vi "USRP Packet Receiver.vi"() -> ()   [LabVIEW 2023]
uses:
  <instrlib>/niUSRP/niUSRP Fetch Rx Data (CDB Cluster).vi
panel:
  out "Sync Found":bool
  out "Correct Packets Rx":i16
  out "Singal & Noise Power":cluster{"signal_power":dbl, "noise_power":dbl}={"signal_power"=1.4546950663593878e-09, "noise_power"=2.571229598792933e-12}
  out "error out":errorcluster={"status"=FALSE, "code"=1074118647, "source"="niUSRP Fetch Rx Data (CDB Cluster).vi<ERR>Overflow: an internal receive buffer has filled before the data could be returned.  Consider reducing the IQ rate, increasing the Fetch rate, or increasing the number of samples per Fetch."}
  in  "Modulation type":string(combo)="QPSK"
  in  "filter parameters":T1={"Alpha"=0.5, "Filter Length"=6, "TX Filter"=enum."Root Raised Cos"} caption="Matching Filter Parameters" {"Alpha" format="%.2f"}
  in  "Acquisition Duration [sec]":dbl=0.04 format="%#.6p"
  out "Actual Rx Parameters":T2={"Rx IQ Sampling\nRate [s/sec]"=200000.0, "Rx Frequency [Hz]"=915000000.0, "Rx Gain [dB]"=20.0, "Rx Antenna"="RX1"} {"Rx Gain [dB]" format="%#.6p"; "Rx Frequency [Hz]" format="%#.6p"; "Rx IQ Sampling\nRate [s/sec]" format="%#.6p"}
  in  "Rx Parameters":T2={"Rx IQ Sampling\nRate [s/sec]"=400000.0, "Rx Frequency [Hz]"=915000000.0, "Rx Gain [dB]"=20.0, "Rx Antenna"="RX1"} {"Rx Gain [dB]" format="%#.6p"; "Rx Frequency [Hz]" format="%#.6p"; "Rx IQ Sampling\nRate [s/sec]" format="%#.6p"}
  in  "USRP IP Address":refnum<k15>="192.168.10.2"
  out "Constellation Graph":T3(graph)
  out "Received Signal (Raw)":dbl[](graph)
  out "Recovered Message":string
  out "Symbol Rate \n[symbols/sec]":dbl=25000.0 format="%#.6p"
  in  "stop":bool
  in  "Continuous Acquire?":bool
  out "Cumulative Packets Recovered":i16(graph)
  out "Signal and Noise Power Tracking":cluster{"total_power":dbl, "noise_power":dbl}(graph)={"total_power"=1.4546950663593878e-09, "noise_power"=2.571229598792933e-12}
  in  "PN Sequence Order for Sync":i32=31
  in  "Packet Parameters":T4={"Guard Bits "=30, "Sync Bits"=20, "Message Bits"=128, "Number of Packets \nto Expect"=46}
  in  "16-PSK System Parameters":T5={"Samples per Symbol"=8, "symbol map"=[], "Differential PSK"=enum."disable", "PSK type"=0} {"PSK type" items=["normal", "shifted", "offset"]; "symbol map" format="%.3f"}
  in  "8-PSK System Parameters":T5={"Samples per Symbol"=8, "symbol map"=[], "Differential PSK"=enum."disable", "PSK type"=0} {"PSK type" items=["normal", "shifted", "offset"]; "symbol map" format="%.3f"}
  in  "QPSK System Parameters":T5={"Samples per Symbol"=8, "symbol map"=[], "Differential PSK"=enum."disable", "PSK type"=0} {"PSK type" items=["normal", "shifted", "offset"]; "symbol map" format="%.3f"}
  in  "BPSK System Parameters":T5={"Samples per Symbol"=8, "symbol map"=[], "Differential PSK"=enum."disable", "PSK type"=0} {"PSK type" items=["normal", "shifted", "offset"]; "symbol map" format="%.3f"}
  in  "synchronization parameters":T6={"expected sync location (symbols)"=-1, "sync sequence"=[], "sync location uncertainty (symbols)"=0, "sync indent (symbols)"=0} {"sync sequence" format="%.2f"}
  # "Guard\nBand"
  # "Sync\nSeq"
  # "Packet\nNumber"
  # "Pad\nData"
  # "Blank\nFrame"
  # "Data"
  # "Packet Receiver"
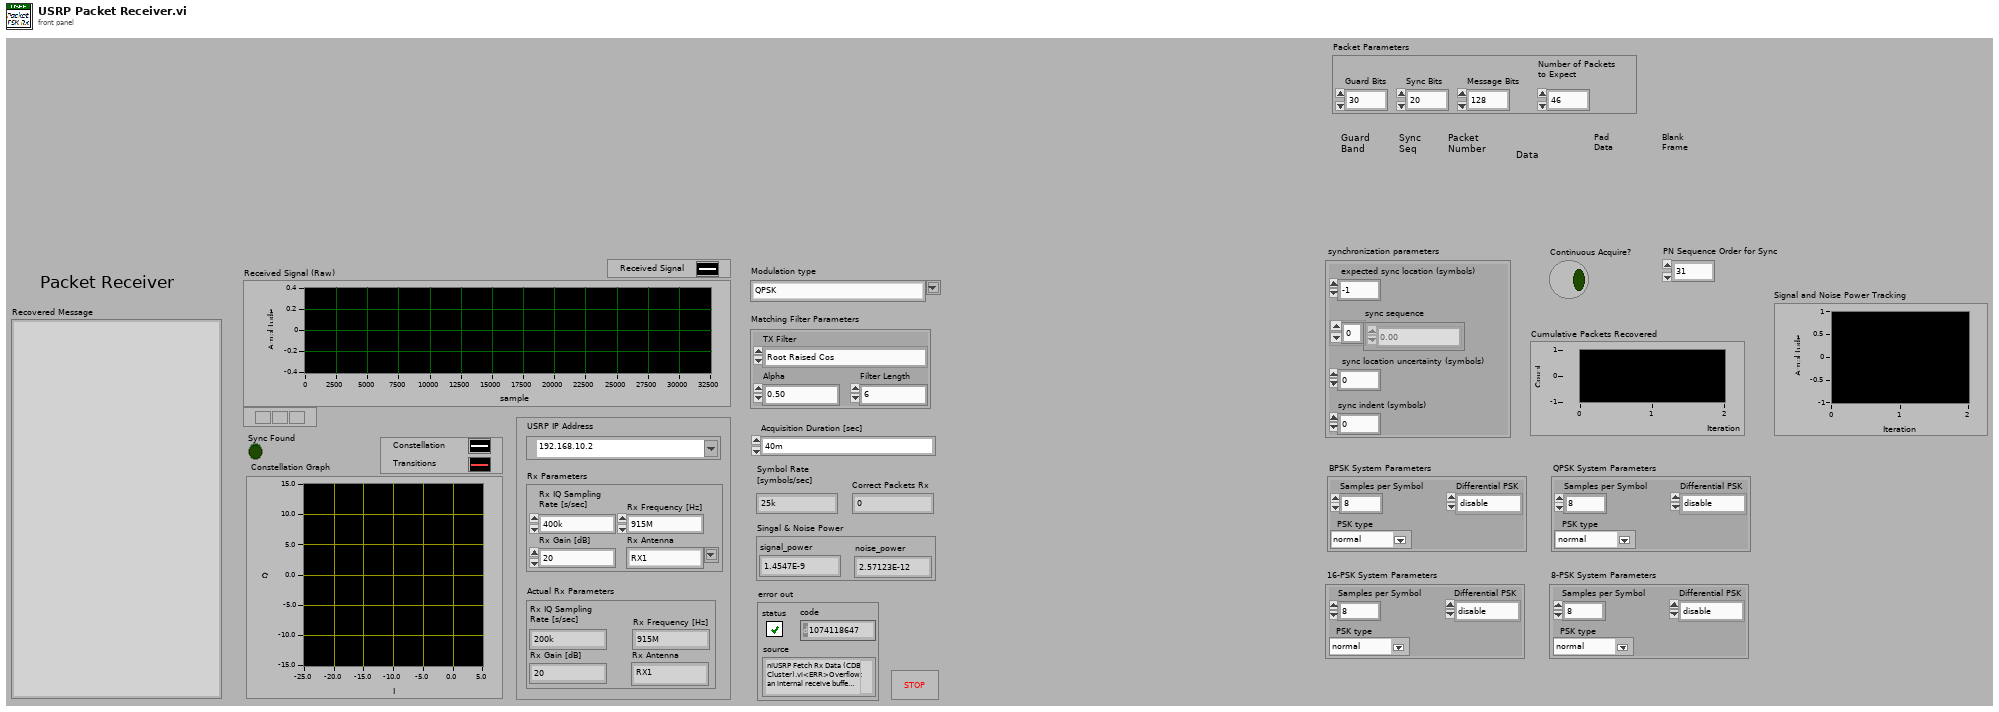
[diagram p1: front panel]
types:
  T1 = cluster{"Alpha":dbl, "Filter Length":i32, "TX Filter":enum16{"none", "Raised Cosine", "Root Raised Cos", "Gaussian"}}
  T2 = cluster{"Rx IQ Sampling\nRate [s/sec]":dbl, "Rx Frequency [Hz]":dbl, "Rx Gain [dB]":dbl, "Rx Antenna":string}
  T3 = cluster{"Decimated Array":dbl[], "Decimated Array":dbl[]}[]
  T4 = cluster{"Guard Bits ":i32, "Sync Bits":i32, "Message Bits":i32, "Number of Packets \nto Expect":i32}
  T5 = cluster{"Samples per Symbol":i32, "symbol map":cdb[], "Differential PSK":enum16{"disable", "enable"}, "PSK type":u16}
  T6 = cluster{"expected sync location (symbols)":i32, "sync sequence":cdb[], "sync location uncertainty (symbols)":i32, "sync indent (symbols)":i32}
  T7 = cluster{"Packet Array":i32[][], "IP Array of Pkt Nums Received  ":bool[]}
  T8 = cluster{"bit stream ":i8[][], "Sync Valid?":bool[], "Decoded Pkt Numbers":u32[], "Enable?":bool}
  T9 = cluster{"packet_arr":cdb[][], "Packets Valid?":bool}
  T10 = cluster{"Rx IQ Sampling\nRate [s/sec]":dbl, "Rx\nFrequency [Hz]":dbl, "Rx Gain [dB]":dbl, "Rx Antenna":string}
  T11 = cluster{"PSK type":u16, "Samples per Symbol":i32, "Differential PSK":enum16{"disable", "enable"}, "M-PSK (4)":i32}
  T12 = cluster{"PSK system parameters":cluster{"samples per symbol (16)":i32, "symbol map":cdb[], "differential PSK":enum16{"disable", "enable"}, "PSK type":u16}, "pulse shaping filter coefficients":dbl[], "matched filter coefficients":dbl[], "synchronization parameters":cluster{"expected sync location (symbols)":i32, "sync sequence":cdb[], "sync location uncertainty (symbols)":i32, "sync indent (symbols)":i32}, "Sync Bits":i8[]}
  T13 = typedef "niAMT.lvlib/Complex Data Waveform.ctl" = cluster{"t0":dbl, "dt":dbl, "Y":cdb[]}
  T14 = cluster{"constellation":dbl[], "oversampled data":dbl[]}[]
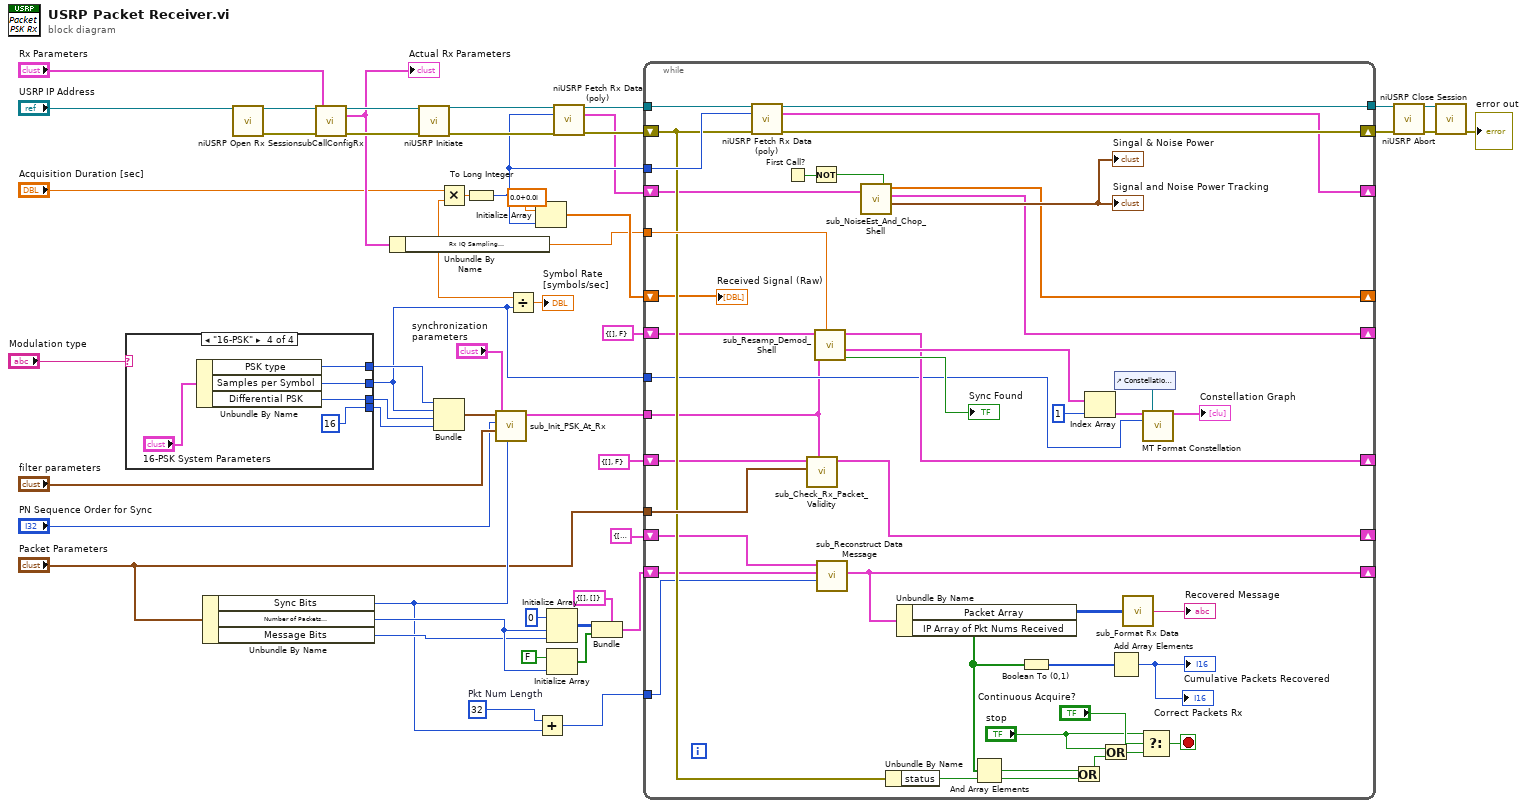
[diagram p0: block diagram]
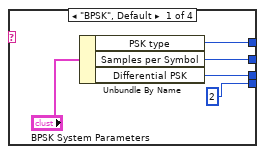
[diagram p2: hidden frame]
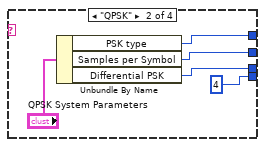
[diagram p3: hidden frame]
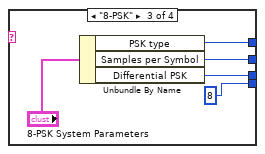
[diagram p4: hidden frame]
diagram:
  w29 = 32  # Pkt Num Length
  n1 = case shown="\"16-PSK\"" "Modulation type" {
    tunnel: [w52 w58 w63 w69] -> w3
    tunnel: [w53 w56 w62 w68] -> w2
    tunnel: [2 ("M-PSK (4)") 4 ("M-PSK (4)") 8 ("M-PSK (4)") 16 ("M-PSK (4)")] -> w1
    tunnel: [w54 w57 w64 w67] -> w4
    frame "BPSK", Default {
      n2 = Unbundle By Name("BPSK System Parameters") -> ("PSK type"=w54:u16, "Samples per Symbol"=w52:i32, "Differential PSK"=w53:enum16{"disable", "enable"})
    }
    frame "QPSK" {
      n3 = Unbundle By Name("QPSK System Parameters") -> ("PSK type"=w57:u16, "Samples per Symbol"=w58:i32, "Differential PSK"=w56:enum16{"disable", "enable"})
    }
    frame "8-PSK" {
      n4 = Unbundle By Name("8-PSK System Parameters") -> ("PSK type"=w64:u16, "Samples per Symbol"=w63:i32, "Differential PSK"=w62:enum16{"disable", "enable"})
    }
    frame "16-PSK" {
      n5 = Unbundle By Name("16-PSK System Parameters") -> ("PSK type"=w67:u16, "Samples per Symbol"=w69:i32, "Differential PSK"=w68:enum16{"disable", "enable"})
    }
  }
  n6 = Unbundle By Name("Packet Parameters") -> ("Sync Bits"=w17:i32, "Number of Packets \nto Expect"=w28:i32, "Message Bits"=w27:i32)
  n7 = call <instrlib>:"niUSRP Open Rx Session.vi"("device names"="USRP IP Address") -> ("session handle out"=w46:refnum<k15>, "error out"=w47:errorcluster)  [unwired: 13 in]
  n8 = call "subCallConfigRx.vi"("session handle"=w46, "Rx Parameters"="Rx Parameters", "error in"=w47) -> ("session handle out"=w44:refnum<k15>, "Actual Rx Parameters"=w30:T10, "error out"=w43:errorcluster)  [unwired: 10 in]
  "Actual Rx Parameters" <- w30
  n9 = Unbundle By Name(w30) -> ("Rx IQ Sampling\nRate [s/sec]"=w6:dbl)
  n10 = call <instrlib>:"niUSRP Initiate.vi"("session handle"=w44, "error in (no error)"=w43) -> ("session handle out"=w13:refnum<k15>, "error out"=w12:errorcluster)  [unwired: 12 in]
  n11 = Bundle("PSK type"=w4, "Samples per Symbol"=w3, "Differential PSK"=w2, "M-PSK (4)"=w1) -> (w34:T11)  [unwired: 1 in]
  n12 = Multiply(x="Acquisition Duration [sec]", y=w6) -> (x*y=w49:dbl)
  n13 = To Long Integer(number=w49) -> (32bit integer=w11:i32)
  n14 = call "sub_Init_PSK_At_Rx.vi"("Sync Bits"=w17, "synchronization parameters"="synchronization parameters", "filter parameters"="filter parameters", "PN sequence order (9)"="PN Sequence Order for Sync", "PSK Parameters"=w34) -> ("PSK Init Parameters"=w33:T12)  [unwired: 5 in, 1 out]
  n15 = Divide(x=w6, y=w3) -> (x/y=→"Symbol Rate \n[symbols/sec]":dbl)
  n16 = Initialize Array(cdb 0.0+0.0i ("element"), w11) -> (w19:cdb[])
  n17 = Add(x=w29, y=w17) -> (x+y=w36:i32)
  n18 = Initialize Array(0, w28, w27) -> (w21:i32[][])
  n19 = Initialize Array(FALSE, w28) -> (w20:bool[])
  n20 = call-poly <instrlib>:"niUSRP Fetch Rx Data (poly).vi"("session handle"=w13, "number of samples"=w11, "error in (no error)"=w12) -> ("session handle out"=w15:refnum<k15>, "data"=w10:cluster{"t0":dbl, "dt":dbl, "Y":cdb[]}, "error out"=w14:errorcluster)  [unwired: 9 in, 1 out]
  n21 = Bundle(cluster=T7 {"Packet Array"=[], "IP Array of Pkt Nums Received  "=[]} ("Packet Info"), "Packet Array"=w21, "IP Array of Pkt Nums Received"=w20) -> (w8:T7)
  n22 = while {
    tunnel: w6 -> [w112]
    tunnel: w15 -> [w94]
    tunnel: [w92] -> w40
    tunnel: w11 -> [w91]
    tunnel: "Packet Parameters" -> [w111]
    tunnel: w36 -> [w78]
    tunnel: w33 -> [w71]
    shift-right: [w93] -> w39
    shift-left: w14 -> [w89]
    tunnel: w3 -> [w72]
    shift-right: [w76] -> _
    shift-left: w8 -> [w79]
    shift-right: [w85] -> _
    shift-left: T9 {"packet_arr"=[], "Packets Valid?"=FALSE} -> [w86]
    shift-right: [w81] -> _
    shift-left: cluster{"bit stream":i8[][], "Enable?":bool} {"bit stream"=[], "Enable?"=FALSE} ("Output Bitstream") -> [w84]
    shift-right: [w70] -> _
    shift-left: T8 {"bit stream "=[], "Sync Valid?"=[], "Decoded Pkt Numbers"=[], "Enable?"=FALSE} ("Output Bit Stream") -> [w80]
    shift-right: [w82] -> _
    shift-left: w10 -> [w83]
    shift-right: [w73] -> _
    shift-left: w19 -> [w74]
    stop <- w107 stop-if-true
    n23 = call-poly <instrlib>:"niUSRP Fetch Rx Data (poly).vi"("session handle"=w94, "number of samples"=w91, "error in (no error)"=w89) -> ("session handle out"=w92:refnum<k15>, "data"=w82:cluster{"t0":dbl, "dt":dbl, "Y":cdb[]}, "error out"=w93:errorcluster)  [unwired: 9 in, 1 out]
    n24 = First Call?() -> (First Call?: T/F=w97:bool)
    n25 = call "sub_Check_Rx_Packet_Validity.vi"("PSK Init Parameters"=w71, "Packet Parameters"=w111, "Input Bit Stream"=w84) -> ("Output Bit Stream"=w70:T8)  [unwired: 7 in]
    n26 = Not(x=w97) -> (.not. x?=w96:bool)
    n27 = call "sub_Resamp_Demod_Shell.vi"("Rx IQ Sampling\nRate [s/sec]"=w112, "PSK Init Parameters"=w71, "Input Packets"=w86) -> ("Synch Found?"=→"Sync Found":bool, "recovered complex waveform"=w100:T13[], "Output Bitstream"=w81:cluster{"bit stream":i8[][], "Enable?":bool})  [unwired: 3 in]
    n28 = call "sub_Reconstruct Data Message.vi"("Start Loc of Data"=w78, "Packet Info"=w79, "Input Stream"=w80) -> ("Packet Info out"=w76:T7)  [unwired: 8 in]
    n29 = call "sub_NoiseEst_And_Chop_Shell.vi"("data"=w83, "Enable"=w96) -> ("Singal & Noise Power"=→"Signal and Noise Power Tracking" →"Singal & Noise Power":cluster{"signal_power":dbl, "noise_power":dbl}, "Output Packets"=w85:cluster{"Packets":cdb[][], "Enable?":bool}, "Delay signal (for plotting use only)"=w73:cdb[])  [unwired: 3 in]
    n30 = Unbundle By Name(w89) -> ("status"=w88:bool)
    n31 = Unbundle By Name(w76) -> ("Packet Array"=w77:i32[][], "IP Array of Pkt Nums Received"=w75:bool[])
    n32 = And Array Elements(Boolean array=w75) -> (logical AND=w90:bool)
    n33 = Boolean To (0,1)(Boolean=w75) -> (0, 1=w110:i16[])
    n34 = Or(x=w90, y=w88) -> (x .or. y?=w87:bool)
    n35 = Index Array(array=w100, index=1) -> (element=w99:T13)
    n36 = Or(x="stop", y=w87) -> (x .or. y?=w108:bool)
    n37 = Add Array Elements(numeric array=w110) -> (sum=→"Correct Packets Rx" →"Cumulative Packets Recovered":i16)
    n38 = control-ref of="Constellation Graph"() -> (w102:refnum<vi>)
    n39 = call "sub_Format Rx Data.vi"("Output Packet Array"=w77) -> ("Received Message"=→"Recovered Message":string)
    n40 = Select(t="stop", s="Continuous Acquire?", f=w108) -> (s? t:f=w107:bool)
    n41 = call <vilib>:"MT Format Constellation.vi"("waveform"=w99, "constellation reference"=w102, "samples per symbol"=w72) -> ("constellation graph"=→"Constellation Graph":T14)  [unwired: 2 in, 10 out]
    "Received Signal (Raw)" <- w74
  }
  n42 = call <instrlib>:"niUSRP Abort.vi"("session handle"=w40, "error in (no error)"=w39) -> ("session handle out"=w41:refnum<k15>, "error out"=w42:errorcluster)  [unwired: 12 in]
  n43 = call <instrlib>:"niUSRP Close Session.vi"("session handle"=w41, "error in (no error)"=w42) -> ("error out"=→"error out":errorcluster)  [unwired: 13 in]
